vi "WithinDist.vi"(6 "Discount start?":bool, 8 "Range":dbl=1.0, 9 "Z":dbl=1.0, 10 "X":dbl=1.0, 11 "All Lines":T1) -> (1 "Index":i32, 2 "In Range?":bool)   [LabVIEW 2014]
uses:
  Libraries/Map Data Folder/All-Lines.ctl
  Libraries/Map Data Folder/LineCluster.ctl
  Libraries/Map Data Folder/LineConnection.ctl
  Libraries/Map Data Folder/Map Data.lvlib
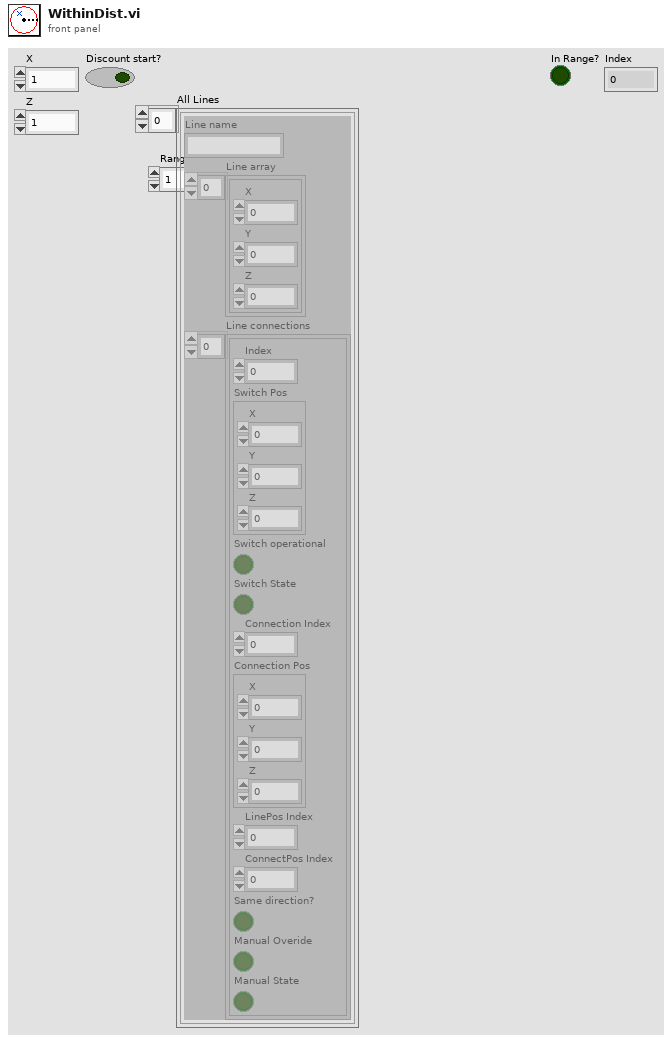
[diagram p1: front panel]
types:
  T1 = typedef "Map Data.lvlib/All-Lines.ctl" = T2[]
  T2 = typedef "Map Data.lvlib/LineCluster.ctl" = cluster{"Line name":string, "Line array":cluster{"X":dbl, "Y":dbl, "Z":dbl}[], "Line connections":T3[]}
  T3 = typedef "LineConnection.ctl" = cluster{"Index":i32, "Switch Pos":cluster{"X":dbl, "Y":dbl, "Z":dbl}, "Switch operational":bool, "Switch State":bool, "Connection Index":i32, "Connection Pos":cluster{"X":dbl, "Y":dbl, "Z":dbl}, "LinePos Index":i32, "ConnectPos Index":i32, "Same direction?":bool, "Manual Overide":bool, "Manual State":bool}
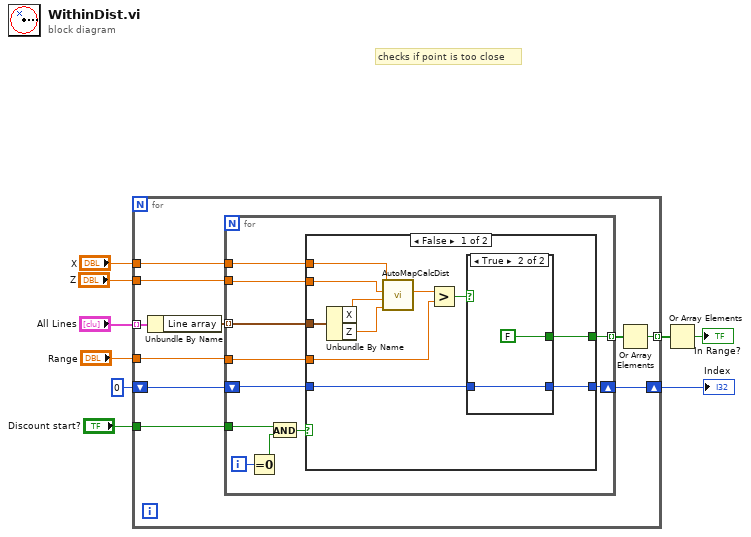
[diagram p0: block diagram]
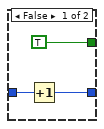
[diagram p2: hidden frame]
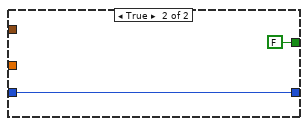
[diagram p3: hidden frame]
diagram:
  # "checks if point is too close"
  n1 = for {
    tunnel: "X" -> [w19]
    tunnel: "Z" -> [w18]
    tunnel: "Range" -> [w17]
    tunnel: [w15] -> w3 mode=indexing
    tunnel: "All Lines" -> [w13] mode=indexing
    shift-right: [w14] -> w6
    shift-left: 0 -> [w11]
    tunnel: "Discount start?" -> [w10]
    n2 = Unbundle By Name(w13) -> ("Line array"=w12:cluster{"X":dbl, "Y":dbl, "Z":dbl}[])
    n3 = for {
      tunnel: w18 -> [w30]
      tunnel: w17 -> [w29]
      tunnel: w12 -> [w28] mode=indexing
      tunnel: [w27] -> w16 mode=indexing
      shift-right: [w25] -> w14
      shift-left: w11 -> [w26]
      tunnel: w19 -> [w24]
      tunnel: w10 -> [w21]
      i -> [w23]
      n4 = Equal To 0?(x=w23) -> (x = 0?=w22:bool)
      n5 = And(x=w21, y=w22) -> (x .and. y?=w20:bool)
      n6 = case shown="False" w20 {
        tunnel: w30 -> [w41 _]
        tunnel: w29 -> [w40 _]
        tunnel: w28 -> [w39 _]
        tunnel: [w38 FALSE] -> w27
        tunnel: w26 -> [w33 w48]
        tunnel: [w32 w48] -> w25
        tunnel: w24 -> [w31 _]
        frame False {
          n7 = Unbundle By Name(w39) -> ("X"=w35:dbl, "Z"=w36:dbl)
          n8 = call "AutoMapCalcDist.vi"("Y2"=w36, "X2"=w35, "Y1"=w41, "X1"=w31) -> ("Distance"=w34:dbl)  [unwired: 7 in]
          n9 = Greater?(x=w34, y=w40) -> (0:w37:bool)
          n10 = case shown="True" w37 {
            tunnel: [TRUE FALSE] -> w38
            tunnel: [w42 w45] -> w32
            tunnel: w33 -> [w43 w45]
            frame False {
              n11 = Increment(x=w43) -> (x+1=w42:i32)
            }
            frame True {
            }
          }
        }
        frame True {
        }
      }
    }
    n12 = Or Array Elements(Boolean array=w16) -> (logical OR=w15:bool)
  }
  "Index" <- w6
  n13 = Or Array Elements(Boolean array=w3) -> (logical OR=→"In Range?":bool)
